vi "GEOM_Amp2Str.vi"(10 "amp":T1={"number"=0, "type"=0, "rotated"=0, "fliped"=0, "FPAcoord"={"xstart"=1, "ystart"=1}, "Physical_size"={"columns"=0, "rows"=0}, "predata"={"columns"=0, "rows"=0}, "postdata"={"columns"=0, "rows"=0}, "Req ROIs"=[], "Corr ROI"=[], "Detnumber"=0, "ampID"="", "discard"=0} {"fliped" items=["none", "horizontal", "vertical"]; "type" items=["LL", "LR", "UL", "UR"]}) -> (2 "resulting string":string)   [LabVIEW 2016]
uses:
  GEOM_AmpType.ctl
  GEOM_Amplifier.ctl
  GEOM_ROI.ctl
  GEOM_Coords.ctl
panel:
  in  "type":T2 items=["LL", "LR", "UL", "UR"]
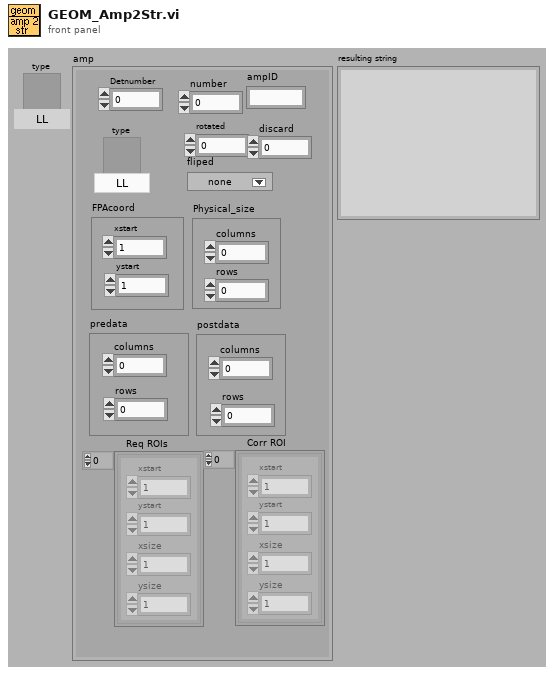
[diagram p1: front panel]
types:
  T1 = typedef "GEOM_Amplifier.ctl" = cluster{"number":i32, "type":T2, "rotated":i16, "fliped":u16, "FPAcoord":cluster{"xstart":i32, "ystart":i32}, "Physical_size":cluster{"columns":i32, "rows":i32}, "predata":cluster{"columns":i32, "rows":i32}, "postdata":cluster{"columns":i32, "rows":i32}, "Req ROIs":T3, "Corr ROI":T3, "Detnumber":i32, "ampID":string, "discard":i32}
  T2 = typedef "GEOM_AmpType.ctl" = u16
  T3 = typedef "GEOM_ROI.ctl" = T4[]
  T4 = typedef "GEOM_Coords.ctl" = cluster{"xstart":u32, "ystart":u32, "xsize":u32, "ysize":u32}
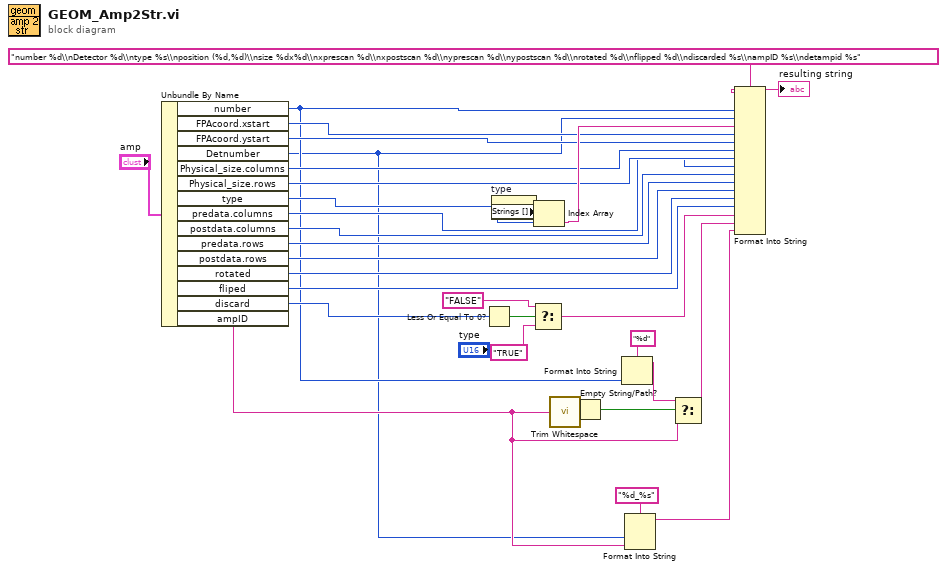
[diagram p0: block diagram]
diagram:
  n1 = Unbundle By Name("amp") -> ("number"=w5:i32, "FPAcoord.xstart"=w26:i32, "FPAcoord.ystart"=w25:i32, "Detnumber"=w1:i32, "Physical_size.columns"=w24:i32, "Physical_size.rows"=w23:i32, "type"=w29:T2, "predata.columns"=w21:i32, "postdata.columns"=w20:i32, "predata.rows"=w19:i32, "postdata.rows"=w18:i32, "rotated"=w17:i16, "fliped"=w16:u16, "discard"=w15:i32, "ampID"=w2:string)
  n2 = Less Or Equal To 0?(x=w15) -> (x <= 0?=w12:bool)
  n3 = property on="type" class="Ring (strict)"() -> ("Strings []"=w30:string[])  [unwired: 2 in, 2 out]
  n4 = Select(t="FALSE", s=w12, f="TRUE") -> (s? t:f=w11:string)
  n5 = Index Array(array=w30, index=w29) -> (element=w27:string)
  n6 = call <vilib>:"Trim Whitespace.vi"("string"=w2) -> ("trimmed string"=w10:string)  [unwired: 1 in]
  n7 = Empty String/Path?(string/path=w10) -> (empty?=w9:bool)
  n8 = Format Into String(format string="%d", w5) -> (resulting string=w7:string)  [unwired: 2 in, 1 out]
  n9 = Format Into String(format string="%d_%s", w1, w2) -> (resulting string=w3:string)  [unwired: 2 in, 1 out]
  n10 = Select(t=w7, s=w9, f=w2) -> (s? t:f=w8:string)
  n11 = Format Into String(format string="number %d\\nDetector %d\\ntype %s\\nposition (%d,%d)\\nsize %dx%d\\nxprescan %d\\nxpostscan %d\\nyprescan %d\\nypostscan %d\\nrotated %d\\nflipped %d\\ndiscarded %s\\nampID %s\\ndetampid %s", w5, w1, w27, w26, w25, w24, w23, w21, w20, w19, w18, w17, w16, w11, w8, w3) -> (resulting string=→"resulting string":string)  [unwired: 2 in, 1 out]
